vi "SensingArea.vi"(0 "Assem Flag":refnum<vi>, 1 "Metal Curr":bool, 2 "Sensing Sw Prev":bool, 4 "Pegs":refnum<vi>, 5 "Peg Flag":refnum<vi>, 7 "Sensing Sw Curr":bool, 9 "RejectionCntrl":refnum<vi>, 12 "Metal Prev":bool, 13 "Plastic Current":bool, 14 "Plastic Previous":bool, 15 "Rings":refnum<vi>) -> ()   [LabVIEW 2016]
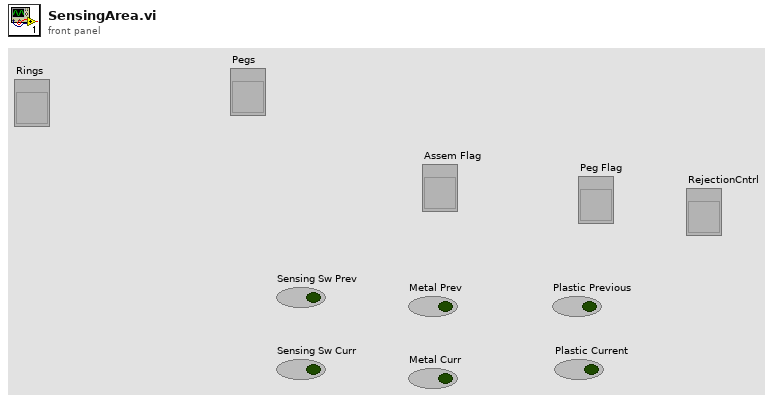
[diagram p1: front panel]
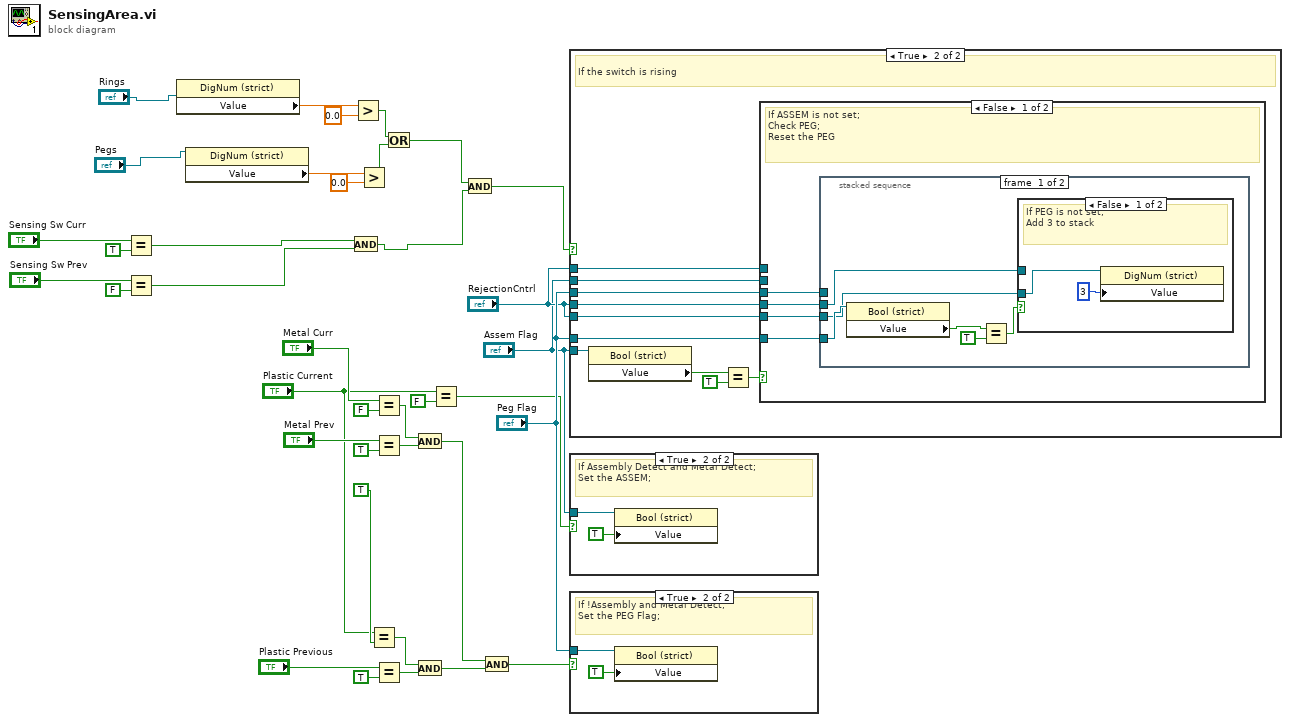
[diagram p0: block diagram]
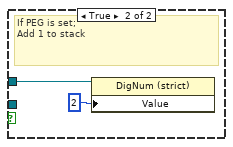
[diagram p3: hidden frame]
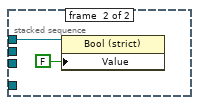
[diagram p4: hidden frame]
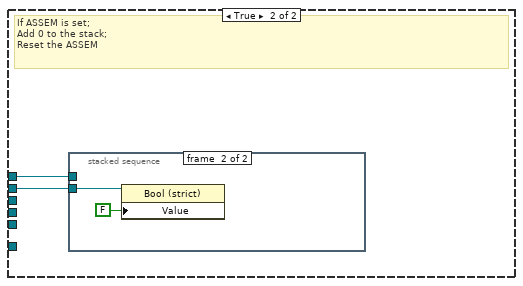
[diagram p5: hidden frame]
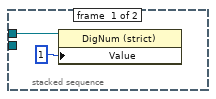
[diagram p6: hidden frame]
diagram:
  n1 = Equal?(x="Sensing Sw Curr", y=TRUE) -> (x = y?=w13:bool)
  n2 = Equal?(x="Sensing Sw Prev", y=FALSE) -> (x = y?=w12:bool)
  n3 = property class="DigNum (strict)"(reference="Rings") -> ("Value"=w9:dbl)  [unwired: 1 in, 2 out]
  n4 = property class="DigNum (strict)"(reference="Pegs") -> ("Value"=w8:dbl)  [unwired: 1 in, 2 out]
  n5 = And(x=w13, y=w12) -> (x .and. y?=w2:bool)
  n6 = Greater?(x=w9, y=0.0) -> (0:w5:bool)
  n7 = Greater?(x=w8, y=0.0) -> (0:w4:bool)
  n8 = Equal?(x="Plastic Current", y=TRUE) -> (x = y?=w27:bool)
  n9 = Equal?(x="Metal Curr", y=FALSE) -> (x = y?=w31:bool)
  n10 = Equal?(x="Metal Prev", y=TRUE) -> (x = y?=w30:bool)
  n11 = Equal?(x="Plastic Previous", y=TRUE) -> (x = y?=w26:bool)
  n12 = Or(x=w5, y=w4) -> (x .or. y?=w3:bool)
  n13 = And(x=w31, y=w30) -> (x .and. y?=w35:bool)
  n14 = And(x=w27, y=w26) -> (x .and. y?=w36:bool)
  n15 = Equal?(x="Plastic Current", y=FALSE) -> (x = y?=w15:bool)
  n16 = And(x=w3, y=w2) -> (x .and. y?=w1:bool)
  n17 = And(x=w35, y=w36) -> (x .and. y?=w37:bool)
  n18 = case shown="True" w1 {
    tunnel: "Assem Flag" -> [_ w44]
    tunnel: "Peg Flag" -> [_ w43]
    tunnel: "RejectionCntrl" -> [_ w42]
    tunnel: "RejectionCntrl" -> [_ w41]
    tunnel: "Peg Flag" -> [_ w40]
    tunnel: "RejectionCntrl" -> [_ w39]
    tunnel: "Assem Flag" -> [_ w38]
    frame False {
      # "Default Operation"
    }
    frame True {
      # "If the switch is rising"
      n19 = property class="Bool (strict)"(reference=w44) -> ("Value"=w47:bool)  [unwired: 1 in, 2 out]
      n20 = Equal?(x=w47, y=TRUE) -> (x = y?=w45:bool)
      n21 = case shown="False" w45 {
        tunnel: w43 -> [w51 _]
        tunnel: w42 -> [w50 _]
        tunnel: w41 -> [w49 _]
        tunnel: w40 -> [w48 _]
        tunnel: w39 -> [_ w65]
        tunnel: w38 -> [_ w64]
        frame False {
          # "If ASSEM is not set;\nCheck PEG;\nReset the PEG"
          n22 = stacked-sequence {
            tunnel: w51 -> [w54 _]
            tunnel: w50 -> [w53 _]
            tunnel: w49 -> [w52 _]
            tunnel: w48 -> [_ w62]
            frame #0 {
              n23 = property class="Bool (strict)"(reference=w54) -> ("Value"=w57:bool)  [unwired: 1 in, 2 out]
              n24 = Equal?(x=w57, y=TRUE) -> (x = y?=w55:bool)
              n25 = case shown="False" w55 {
                tunnel: w53 -> [w58 _]
                tunnel: w52 -> [_ w60]
                frame False {
                  # "If PEG is not set;\nAdd 3 to stack"
                  n26 = property class="DigNum (strict)"(reference=w58, "Value"=i8 3 ("Rejection Control")) -> ()  [unwired: 1 in, 2 out]
                }
                frame True {
                  # "If PEG is set;\nAdd 1 to stack"
                  n27 = property class="DigNum (strict)"(reference=w60, "Value"=i8 2 ("Rejection Control")) -> ()  [unwired: 1 in, 2 out]
                }
              }
            }
            frame #1 {
              n28 = property class="Bool (strict)"(reference=w62, "Value"=FALSE ("Peg Flag")) -> ()  [unwired: 1 in, 2 out]
            }
          }
        }
        frame True {
          # "If ASSEM is set;\nAdd 0 to the stack;\nReset the ASSEM"
          n29 = stacked-sequence {
            tunnel: w65 -> [w66 _]
            tunnel: w64 -> [_ w68]
            frame #0 {
              n30 = property class="DigNum (strict)"(reference=w66, "Value"=i8 1 ("Rejection Control")) -> ()  [unwired: 1 in, 2 out]
            }
            frame #1 {
              n31 = property class="Bool (strict)"(reference=w68, "Value"=FALSE ("Assembly Flag")) -> ()  [unwired: 1 in, 2 out]
            }
          }
        }
      }
    }
  }
  n32 = case shown="True" w15 {
    tunnel: "Assem Flag" -> [_ w70]
    frame False {
    }
    frame True {
      # "If Assembly Detect and Metal Detect;\nSet the ASSEM;"
      n33 = property class="Bool (strict)"(reference=w70, "Value"=TRUE ("Assembly Flag")) -> ()  [unwired: 1 in, 2 out]
    }
  }
  n34 = case shown="True" w37 {
    tunnel: "Peg Flag" -> [_ w72]
    frame False {
    }
    frame True {
      # "If !Assembly and Metal Detect;\nSet the PEG Flag;"
      n35 = property class="Bool (strict)"(reference=w72, "Value"=TRUE ("Peg Flag")) -> ()  [unwired: 1 in, 2 out]
    }
  }
